vi "Data_Array_To_Decimal.vi"(0 "Data_Erd_Read":string[](array[string])) -> (4 "Data_Decimal":string[](array[string]))   [LabVIEW 2023]
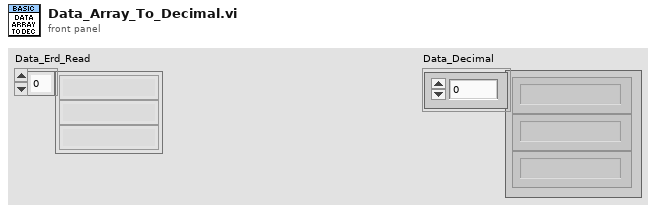
[diagram p1: front panel]
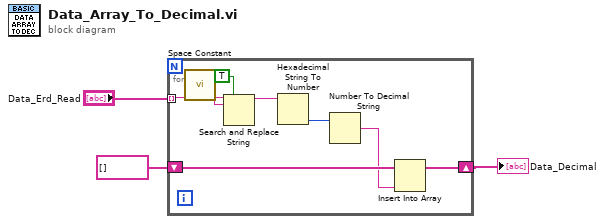
[diagram p0: block diagram]
diagram:
  n1 = for {
    tunnel: "Data_Erd_Read" -> [w6] mode=indexing
    shift-right: [w9] -> w1
    shift-left: string[] [] -> [w10]
    n2 = call <vilib>:"Space Constant.vi"() -> ("String"=w5:string)
    n3 = Search and Replace String(replace all?=TRUE ("replace all? (F)"), input string=w6, search string=w5) -> (result string=w7:string)  [unwired: 5 in, 3 out]
    n4 = Hexadecimal String To Number(string=w7) -> (number=w11:u32)  [unwired: 2 in, 1 out]
    n5 = Number To Decimal String(number=w11) -> (decimal integer string=w8:string)  [unwired: 1 in]
    n6 = Insert Into Array(array=w10, new element=w8) -> (w9:string[])  [unwired: 1 in]
  }
  "Data_Decimal" <- w1
